vi "RageATE-LightBar.vi"(0 "VISA resource name":refnum<visa-resource-name>, 11 "error in":errorcluster, 12 "Select":u32(ring) items=["OFF"=0, "RED"=1, "AMBER"=2, "GREEN"=4, "GRE+AMBER"=6, "ALL"=7, "BUZZ"=8, "RED+BUZZ"=9, "ALL+BUZZ"=15], 13 "RO(T)":bool) -> (3 "Read":u32, 4 "VISA resource name out":refnum<visa-resource-name>, 15 "error out":errorcluster)   [LabVIEW 2018]
uses:
  Zaber A Series.lvlib
panel:
  out "W=R?(T)":bool[](array[boolean])
  out "Boolean array":bool[](array[boolean])
  in  "RED":bool
  in  "GREEN":bool
  in  "AMBER":bool
  in  "BUZZER":bool
  out "Digital Output 1":bool
  out "Digital Output 2":bool
  out "Digital Output 3":bool
  out "Digital Output 4":bool
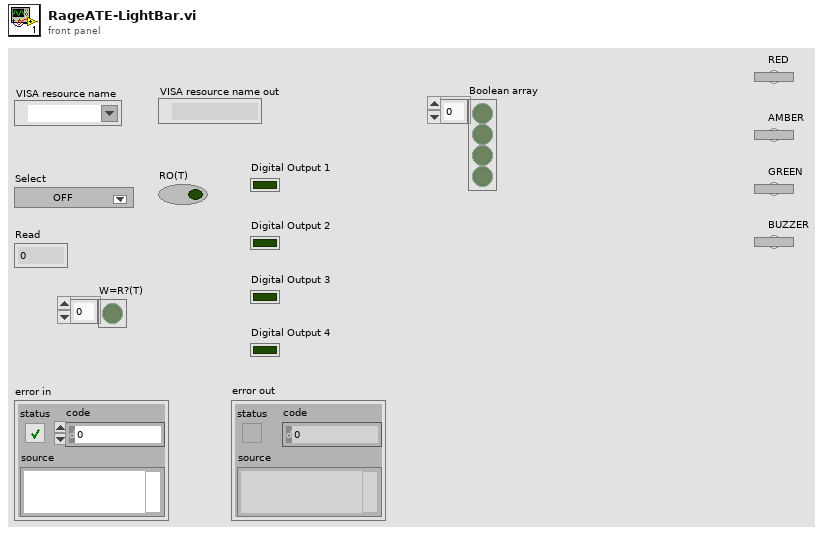
[diagram p1: front panel]
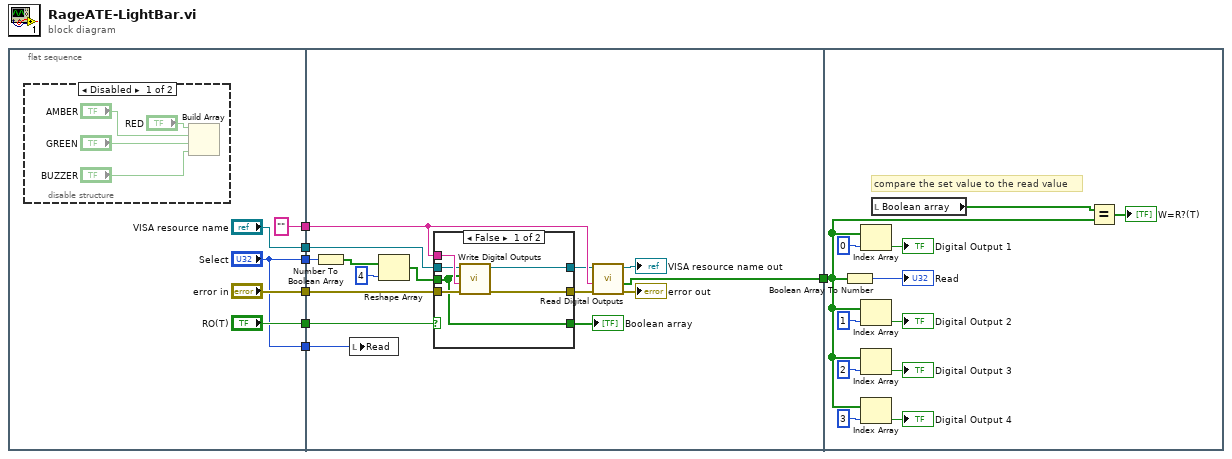
[diagram p0: block diagram]
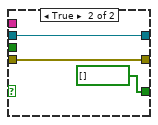
[diagram p3: hidden frame]
diagram:
  n1 = flat-sequence {
    tunnel: ["" ("Device Number")] -> w7
    tunnel: ["error in"] -> w6
    tunnel: ["VISA resource name"] -> w5
    tunnel: ["Select"] -> w3
    tunnel: ["RO(T)"] -> w2
    tunnel: ["Select"] -> w1
    tunnel: [w26] -> w4
    tunnel: w5 -> [w22]
    tunnel: w6 -> [w23]
    tunnel: w7 -> [w31]
    tunnel: w3 -> [w19]
    tunnel: w2 -> [w18]
    tunnel: w1 -> [w17]
    tunnel: w4 -> [w42]
    frame #0 {
      n2 = disable-structure shown="Disabled" {
        frame Disabled {
          n3 = Build Array("RED", "AMBER", "GREEN", "BUZZER") -> ()  [unwired: 1 out]
        }
        frame Enabled {
        }
      }
    }
    frame #1 {
      n4 = Number To Boolean Array(number=w19) -> (Boolean array=w21:bool[])
      n5 = local write "Read"(w17) -> ()
      n6 = Reshape Array(w21, 4 ("dimension size")) -> (w25:bool[])
      n7 = case shown="False" w18 {
        tunnel: w31 -> [w37 _]
        tunnel: [w36 w39] -> w29
        tunnel: [w35 w40] -> w28
        tunnel: w25 -> [w32 _]
        tunnel: w23 -> [w34 w39]
        tunnel: w22 -> [w33 w40]
        tunnel: [w32 bool[] [] ("Boolean array")] -> w20
        frame False {
          n8 = call "Write Digital Outputs.vi"("error in (no error)"=w34, "Device Number"=w37, "Digital Outputs"=w32, "VISA resource name"=w33) -> ("error out"=w36:errorcluster, "VISA resource name out"=w35:refnum<visa-resource-name>)  [unwired: 6 in]
        }
        frame True {
        }
      }
      "Boolean array" <- w20
      n9 = call "Read Digital Outputs.vi"("error in (no error)"=w29, "Device Number"=w31, "VISA resource name"=w28) -> ("error out"=→"error out":errorcluster, "Digital Output Pins"=w26:bool[], "VISA resource name out"=→"VISA resource name out":refnum<visa-resource-name>)  [unwired: 6 in]
    }
    frame #2 {
      # "compare the set value to the read value"
      n10 = Boolean Array To Number(Boolean array=w42) -> (number=→"Read":u32)
      n11 = Index Array(array=w42, index=0) -> (element=→"Digital Output 1":bool)
      n12 = Index Array(array=w42, index=1) -> (element=→"Digital Output 2":bool)
      n13 = Index Array(array=w42, index=2) -> (element=→"Digital Output 3":bool)
      n14 = Index Array(array=w42, index=3) -> (element=→"Digital Output 4":bool)
      n15 = local read "Boolean array"() -> (w44:bool[])
      n16 = Equal?(x=w44, y=w42) -> (x = y?=→"W=R?(T)":bool[])
    }
  }
